vi "Set Configuration.vi"(8 "error in":errorcluster, 10 "transfer settings":T1, 11 "RDMA Transfer Tx Configuration in":refnum<class "RDMA Transfer Tx Configuration.lvclass">) -> (0 "error out":errorcluster, 3 "RDMA Transfer Tx Configuration out":refnum<class "RDMA Transfer Tx Configuration.lvclass">)   [LabVIEW 2020, in "RDMA.lvlib" / "RDMA Transfer Tx Configuration.lvclass"]
uses:
  RDMA Transfer Tx Configuration.lvclass
  Tx Transfer Settings.ctl
  RDMA Transfer Tx Configuration.lvclass/RDMA Transfer Tx Configuration.ctl
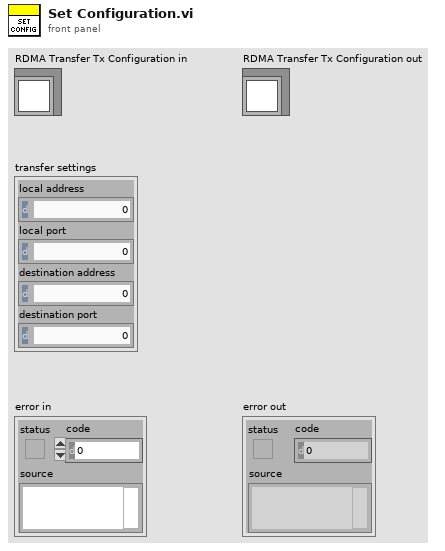
[diagram p1: front panel]
types:
  T1 = typedef "RDMA.lvlib/RDMA Transfer Tx Configuration.lvclass/Tx Transfer Settings.ctl" = cluster{"local address":u32, "local port":u16, "destination address":u32, "destination port":u16}
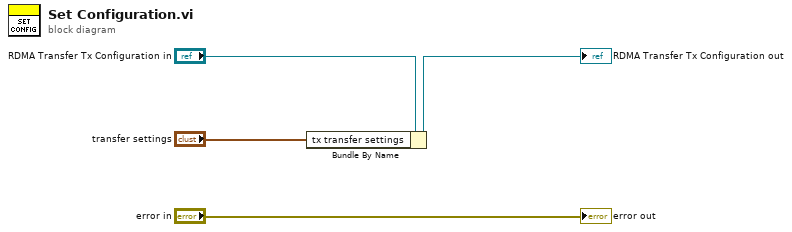
[diagram p0: block diagram]
diagram:
  n1 = Bundle By Name(cluster="RDMA Transfer Tx Configuration in", "tx transfer settings"="transfer settings") -> (→"RDMA Transfer Tx Configuration out":refnum<class "RDMA Transfer Tx Configuration.lvclass">)
  "error out" <- "error in"
